vi "http read headers from stream.vi"(8 "error in":errorcluster, 9 "max header size":i32, 10 "timeout ms":i32, 11 "TCP Network Connection in":refnum<k5>) -> (0 "error out":errorcluster, 3 "headers":T1)   [LabVIEW 2013, in "http headers.lvlib"]
uses:
  http headers.lvlib
  http header data.ctl
  <vilib>/dlg_ctls.llb/Space Constant.vi
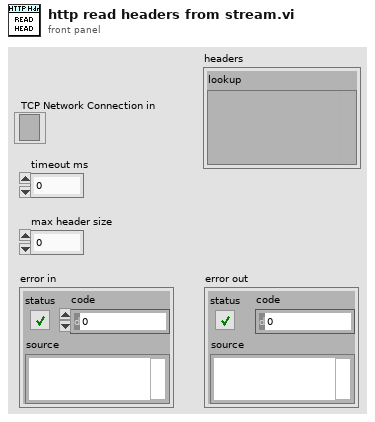
[diagram p1: front panel]
types:
  T1 = typedef "http headers.lvlib/http header data.ctl" = cluster{"lookup":variant}
  T2 = enum16{"Standard", "Buffered", "CRLF", "Immediate"}
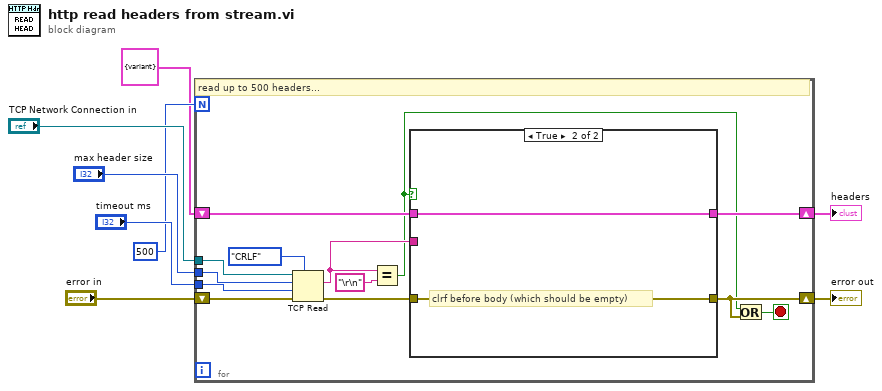
[diagram p0: block diagram]
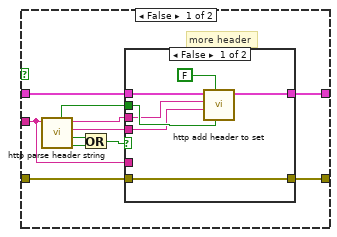
[diagram p2: hidden frame]
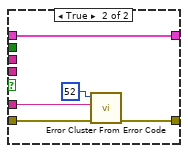
[diagram p3: hidden frame]
diagram:
  n1 = for {
    N: 500 -> [_]
    tunnel: "TCP Network Connection in" -> [w20]
    tunnel: "max header size" -> [w19]
    tunnel: "timeout ms" -> [w18]
    shift-right: [w12] -> w2
    shift-left: "error in" -> [w17]
    shift-right: [w15] -> w1
    shift-left: T1 {"lookup"=variant} ("headers") -> [w16]
    stop <- w10 stop-if-true
    # "read up to 500 headers..."
    n2 = TCP Read(connection ID=w20, bytes to read=w19, error in (no error)=w17, 7:T2."CRLF" ("mode (standard)"), 9:w18) -> (data out=w13:string, error out=w14:errorcluster)  [unwired: 1 out]
    n3 = Equal?(x=w13, y="\r\n" ("x")) -> (x = y?=w9:bool)
    n4 = case shown="True" w9 {
      tunnel: w16 -> [w32 w45]
      tunnel: [w31 w45] -> w15
      tunnel: w14 -> [w27 w46]
      tunnel: w13 -> [w22 _]
      tunnel: [w23 w46] -> w12
      frame False {
        # "more header"
        n5 = call "http parse header string.vi"("raw string"=w22) -> ("no field name"=w24:bool, "no crlf"=w26:bool, "header field data"=w28:string, "header field name"=w29:string, "continuation"=w30:bool)  [unwired: 6 in]
        n6 = Or(x=w26, y=w24) -> (x .or. y?=w25:bool)
        n7 = case shown="False" w25 {
          tunnel: w32 -> [w39 w42]
          tunnel: [w38 w42] -> w31
          tunnel: w30 -> [w36 _]
          tunnel: w29 -> [w35 _]
          tunnel: w28 -> [w34 _]
          tunnel: [w33 w43] -> w23
          tunnel: w27 -> [w33 w44]
          tunnel: w22 -> [_ w40]
          frame False {
            n8 = call "http add header to set.vi"("continuation?"=w36, "override on duplicate?"=FALSE, "header field data"=w34, "header field name"=w35, "headers in"=w39) -> ("headers out"=w38:T1)  [unwired: 6 in]
          }
          frame True {
            n9 = call <vilib>:"Error Cluster From Error Code.vi"("error in (no error)"=w44, "error message (\"\")"=w40, "error code (0)"=52) -> ("error out"=w43:errorcluster)  [unwired: 6 in]
          }
        }
      }
      frame True {
        # "clrf before body (which should be empty)"
      }
    }
    n10 = Or(x=w9, y=w12) -> (x .or. y?=w10:bool)
  }
  "error out" <- w2
  "headers" <- w1
